vi "Read Temperature.vi"(0 "device session in":refnum<class "Device Session.lvclass">, 5 "source":T1, 11 "error in":errorcluster) -> (4 "device session out":refnum<class "Device Session.lvclass">, 6 "temperature (°C)":dbl, 15 "error out":errorcluster)   [LabVIEW 2021, in "Device Session.lvclass"]
doc: "Returns a specified temperature measurement, in degrees Celsius.\n\n<B>Input Parameters</B>\n\n<B>device session in</B> is a reference to the Device Session object, which contains a session to each instrument design library used in this sample project. This parameter is obtained from the 'Open Session' VI.\n\n<B>source</B> specifies the source of the temperature measurement to be returned by the 'temperature' output.\n\n'Device Temperature': specifies the temperature of the analog front-end of the device as the temperature to return.\n'Thermal Shutdown Margin': specifies the temperature difference between the FPGA temperature sensor and the FPGA temperature limit as the measurement to return.\n'FPGA Temperature': specifies the current FPGA die temperature as the measurement to return.\n'FPGA Temperature Limit': specifies the thermal shutdown limit of the FPGA sensor as the measurement to return.\n\n<B>error in</B> describes error conditions that occur before this node runs. This input provides standard 'error in' functionality.\n\n<B>Output Parameters</B>\n\n<B>device session out</B> passes a reference to the session to the next VI.\n\n<B>temperature (°C)</B> returns the temperature measurement in degrees Celsius.\n\n<B>error out</B> contains error information. This output provides standard 'error out' functionality."
uses:
  Device Session.lvclass
  <instrlib>/HSAI-RIO/Types/v1/Host/Typedefs/Temp Source.ctl
  Device Session.lvclass/Device Session.ctl
  <instrlib>/HSAI-RIO/Config/Group A/v1/Host/Main/niHSAI Group A Config v1 Host.lvclass
  <instrlib>/HSAI-RIO/Types/v1/Host/niHSAI Types v1 Host.lvlib
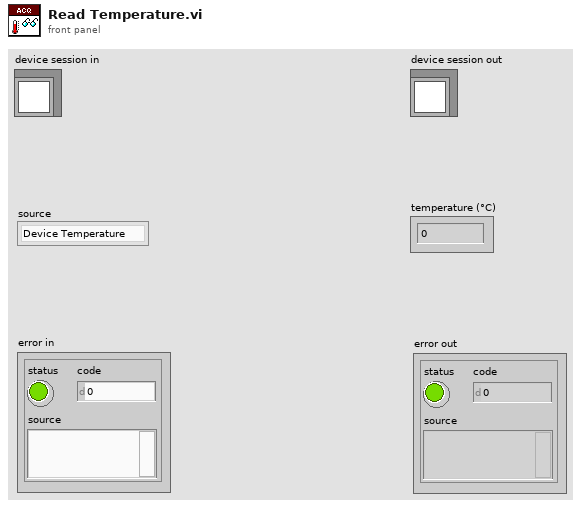
[diagram p1: front panel]
types:
  T1 = typedef "niHSAI Types v1 Host.lvlib/Temp Source.ctl" = enum8{"Device Temperature", "Thermal Shutdown Margin", "FPGA Temperature", "FPGA Temperature Limit"}
  T2 = typedef "Device Session.lvclass/Device Session Object.ctl" = cluster{"fpga reference":T3, "reg bus":refnum<class "niInstr FIFO Register Bus v1 Host.lvclass">, "subsystem map":refnum<class "niInstr Subsystem Map v1 Host.lvclass">, "cal data":refnum<class "niHSAI Cal Data v1 Host.lvclass">, "config":refnum<class "niHSAI Group A Config v1 Host.lvclass">, "acquisition 0":refnum<class "niInstr Multirecord Acquisition v1 Host.lvclass">, "acquisition 1":refnum<class "niInstr Multirecord Acquisition v1 Host.lvclass">, "acquisition 2":refnum<class "niInstr Multirecord Acquisition v1 Host.lvclass">, "acquisition 3":refnum<class "niInstr Multirecord Acquisition v1 Host.lvclass">, "acquisition 4":refnum<class "niInstr Multirecord Acquisition v1 Host.lvclass">, "acquisition 5":refnum<class "niInstr Multirecord Acquisition v1 Host.lvclass">, "acquisition 6":refnum<class "niInstr Multirecord Acquisition v1 Host.lvclass">, "acquisition 7":refnum<class "niInstr Multirecord Acquisition v1 Host.lvclass">, "number of selected acq channels":u8, "selected acq channels":bool[], "number of channels":u32, "configured channels":bool[], "acq configuration":cluster{"number of samples":u64, "number of records":u64, "pretrigger samples":u64}, "actual channel configuration":T4[], "sample clock rate (Hz)":dbl, "scaling coefficients":T8[]}
  T3 = typedef "Device Session.lvclass/FPGA Refnum.ctl" = refnum<k20>
  T4 = typedef "niHSAI Types v1 Host.lvlib/Channel Configuration.ctl" = cluster{"channel":u32, "coupling":T5, "impedance":T6, "bandwidth":T7, "vertical range":dbl, "vertical offset":dbl}
  T5 = typedef "niHSAI Types v1 Host.lvlib/Coupling.ctl" = enum8{"Default", "DC", "AC"}
  T6 = typedef "niHSAI Types v1 Host.lvlib/Impedance.ctl" = enum8{"Default", "1 mega ohm", "50 ohm"}
  T7 = typedef "niHSAI Types v1 Host.lvlib/Bandwidth.ctl" = enum8{"Default", "Full Bandwidth", "Anti-alias Filter", "150 MHz"}
  T8 = typedef "niInstr Multirecord Acquisition v1 Host.lvclass/Scaling Coefficient.ctl" = cluster{"gain":dbl, "offset":dbl}
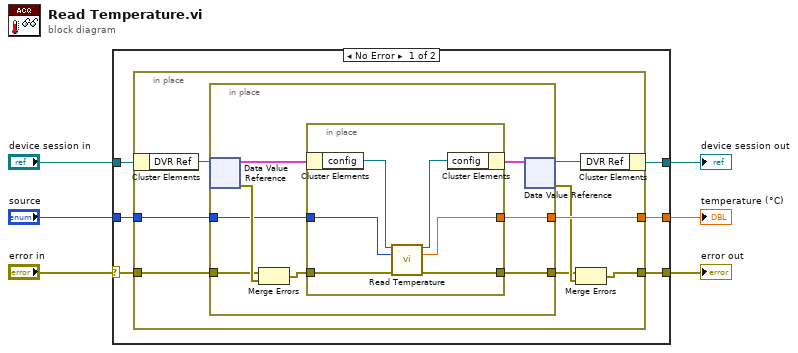
[diagram p0: block diagram]
diagram:
  n1 = case shown="No Error" "error in" {
    selector: "error in" -> [w12 w36]
    tunnel: [w9 w36] -> w5
    tunnel: [w7 w35] -> w4
    tunnel: "device session in" -> [w8 w35]
    tunnel: [w11 _] -> w2
    tunnel: "source" -> [w10 _]
    frame No Error {
      n2 = in-place {
        in-place-border: w12 -> [w20]
        in-place-border: [w19] -> w11
        in-place-border: w10 -> [w16]
        in-place-border: [w15] -> w9
        n3 = in-place-cluster #1(w8) -> ("DVR Ref"=w14:refnum<data-value>)
        n4 = in-place {
          in-place-border: w20 -> [w26]
          in-place-border: [w24] -> w19
          in-place-border: [w27] -> w17
          in-place-border: w16 -> [w25]
          n5 = in-place-dvr #2(w14) -> (w22:T2, w28:errorcluster)
          n6 = Merge Errors(w26, w28) -> (w23:errorcluster)
          n7 = in-place {
            in-place-border: [w34] -> w27
            in-place-border: w23 -> [w33]
            in-place-border: w25 -> [w32]
            in-place-border: [w31] -> w24
            n8 = in-place-cluster #3(w22) -> ("config"=w30:refnum<class "niHSAI Group A Config v1 Host.lvclass">)
            n9 = call-dynamic "Read Temperature.vi"("session in"=w30, "source"=w32, "error in"=w33) -> ("session out"=w29:refnum<class "niHSAI Group A Config v1 Host.lvclass">, "temperature (°C)"=w31:dbl, "error out"=w34:errorcluster)  [unwired: 10 in]
            n10 = in-place-cluster #3("config"=w29) -> (w21:T2)
          }
          n11 = in-place-dvr #2(w21) -> (w13:refnum<data-value>, w18:errorcluster)
        }
        n12 = Merge Errors(w17, w18) -> (w15:errorcluster)
        n13 = in-place-cluster #1("DVR Ref"=w13) -> (w7:refnum<class "Device Session.lvclass">)
      }
    }
    frame Error {
    }
  }
  "error out" <- w5
  "device session out" <- w4
  "temperature (°C)" <- w2
